vi "properties.set.vi"(8 "error in":errorcluster, 10 "Properties":refnum<class "properties.lvclass">, 11 "asset in":refnum<class "asset.lvclass">) -> (0 "error out":errorcluster, 3 "asset out":refnum<class "asset.lvclass">)   [LabVIEW 2020, in "asset.lvclass"]
uses:
  asset.lvclass
  asset.lvclass/asset.ctl
  Nominal Client/Nominal Client.lvclass
  nominal types/properties/properties.lvclass
  <vilib>/JDP Science/JSONtext/JSONtext.lvlib
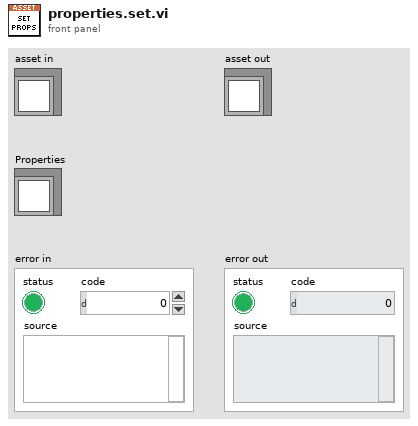
[diagram p1: front panel]
types:
  T1 = typedef "dataScopes.lvlib/links.ctl" = cluster{"URL":string, "Title":string}[]
  T2 = typedef "dataScopes.lvlib/data_scopes.ctl" = T3[]
  T3 = typedef "dataScopes.lvlib/data_scope.ctl" = cluster{"dataScopeName":string, "dataSource":T4, "seriesTags":refnum<class "properties.lvclass">, "offset":T6}
  T4 = typedef "dataScopes.lvlib/data_source.ctl" = cluster{"type":T5, "rid":string}
  T5 = typedef "dataScopes.lvlib/type.ctl" = enum16{"dataset", "connection", "logSet", "video"}
  T6 = typedef "dataScopes.lvlib/offset.ctl" = cluster{"seconds":i32, "nanos":i32, "picos":i32}
  T7 = cluster{"rid":string, "title":string, "properties":refnum<class "properties.lvclass">, "labels":refnum<class "labels.lvclass">, "Links":T1, "datascopes":T2, "createdAt":timestamp, "updatedAt":timestamp, "attachments":refnum<class "labels.lvclass">, "isStaged":bool, "isArchived":bool, "description":string, "createdBy":string, "type":string}
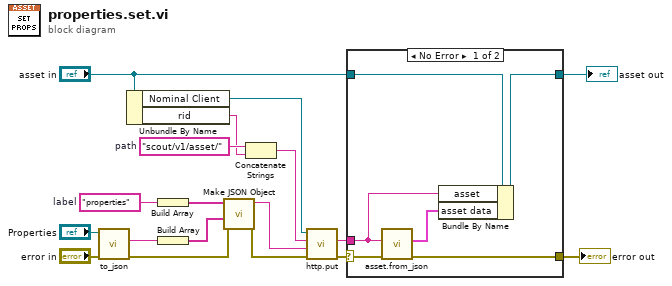
[diagram p0: block diagram]
diagram:
  w4 = "properties"  # label
  w17 = "scout/v1/asset/"  # path
  n1 = call-dynamic "to_json.vi"("error in"="error in", "properties in"="Properties") -> ("error out"=w1:errorcluster, "json"=w7:string)  [unwired: 6 in, 2 out]
  n2 = Unbundle By Name("asset in") -> ("Nominal Client"=w18:refnum<class "Nominal Client.lvclass">, "rid"=w15:string)
  n3 = Build Array(w4) -> (w5:string[])
  n4 = Build Array(w7) -> (w6:string[])
  n5 = call <vilib>:"Make JSON Object.vi"("error in (no error)"=w1, "JSON Items"=w6, "Item Names"=w5) -> ("error out"=w2:errorcluster, "<JSON>"=w3:string)  [unwired: 7 in]
  n6 = Concatenate Strings(w17, w15) -> (w16:string)
  n7 = call "http.put.vi"("error in"=w2, "Body"=w3, "Path"=w16, "Nominal Client in"=w18) -> ("error out"=w14:errorcluster, "Response"=w11:string)  [unwired: 4 in, 2 out]
  n8 = case shown="No Error" w14 {
    selector: w14 -> [w24 w26]
    tunnel: [w23 w26] -> w13
    tunnel: "asset in" -> [w22 w25]
    tunnel: w11 -> [w20 _]
    tunnel: [w19 w25] -> w10
    frame No Error {
      n9 = call "asset.from_json.vi"("error in"=w24, "asset"=w20) -> ("error out"=w23:errorcluster, "Asset Data"=w21:T7)  [unwired: 8 in]
      n10 = Bundle By Name(cluster=w22, "asset"=w20, "asset data"=w21) -> (w19:refnum<class "asset.lvclass">)
    }
    frame Error {
    }
  }
  "asset out" <- w10
  "error out" <- w13
